vi "Flush if true.vi"(8 "error in":errorcluster, 10 "Bytes at port > X":bool, 11 "port in":refnum<visa-resource-name>) -> (0 "error out":errorcluster, 3 "port out":refnum<visa-resource-name>)   [LabVIEW 2013]
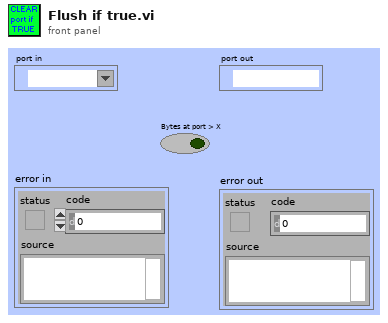
[diagram p1: front panel]
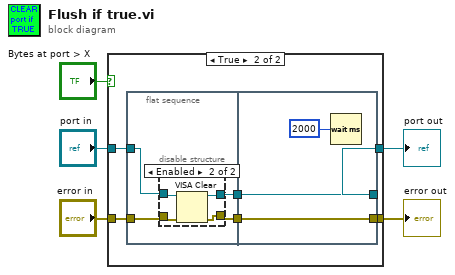
[diagram p0: block diagram]
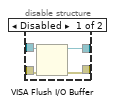
[diagram p3: hidden frame]
diagram:
  n1 = case shown="True" "Bytes at port > X" {
    tunnel: [w7 w13] -> w1
    tunnel: "error in" -> [w7 w11]
    tunnel: "port in" -> [w6 w10]
    tunnel: [w6 w8] -> w5
    frame False {
    }
    frame True {
      n2 = flat-sequence {
        tunnel: [w17] -> w12
        tunnel: w11 -> [w16]
        tunnel: w10 -> [w14]
        tunnel: [w15] -> w9
        tunnel: [w27] -> w13
        tunnel: w12 -> [w27]
        tunnel: [w26] -> w8
        tunnel: w9 -> [w26]
        frame #0 {
          n3 = disable-structure shown="Enabled" {
            disable-tunnel: [w21 w22] -> w17
            disable-tunnel: w16 -> [w20 w25]
            disable-tunnel: [w19 w23] -> w15
            disable-tunnel: w14 -> [w18 w24]
            frame Disabled {
              n4 = VISA Flush I/O Buffer(VISA resource name=w18, error in (no error)=w20) -> (VISA resource name out=w19:refnum<visa-resource-name>, error out=w21:errorcluster)  [unwired: 1 out]
            }
            frame Enabled {
              n5 = VISA Clear(VISA resource name=w24, error in (no error)=w25) -> (VISA resource name out=w23:refnum<visa-resource-name>, error out=w22:errorcluster)
            }
          }
        }
        frame #1 {
          n6 = Wait (ms)(milliseconds to wait=u32 2000) -> ()  [unwired: 1 out]
        }
      }
    }
  }
  "port out" <- w5
  "error out" <- w1
